vi "Generic Request (File).vi"(5 "method":string, 6 "timeout":i32=10000, 7 "output file":path, 8 "error in":errorcluster, 9 "file":path, 10 "url":string, 11 "Session In":refnum<class "Session.lvclass">) -> (0 "error out":errorcluster, 1 "body":string, 2 "headers":string, 3 "Session Out":refnum<class "Session.lvclass">, 4 "status code":u32)   [LabVIEW 2020, in "Library Commun.lvlib" / "Library Http.lvlib" / "Session.lvclass"]
uses:
  Session.lvclass
  Session.lvclass/Session.ctl
  lvwebclient_32.dll
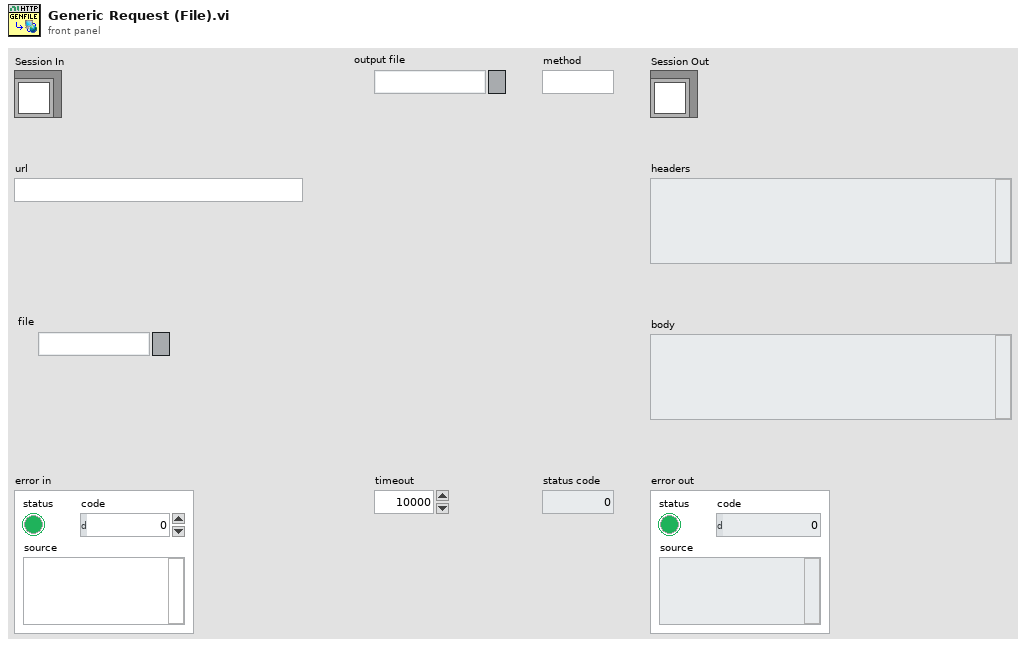
[diagram p1: front panel]
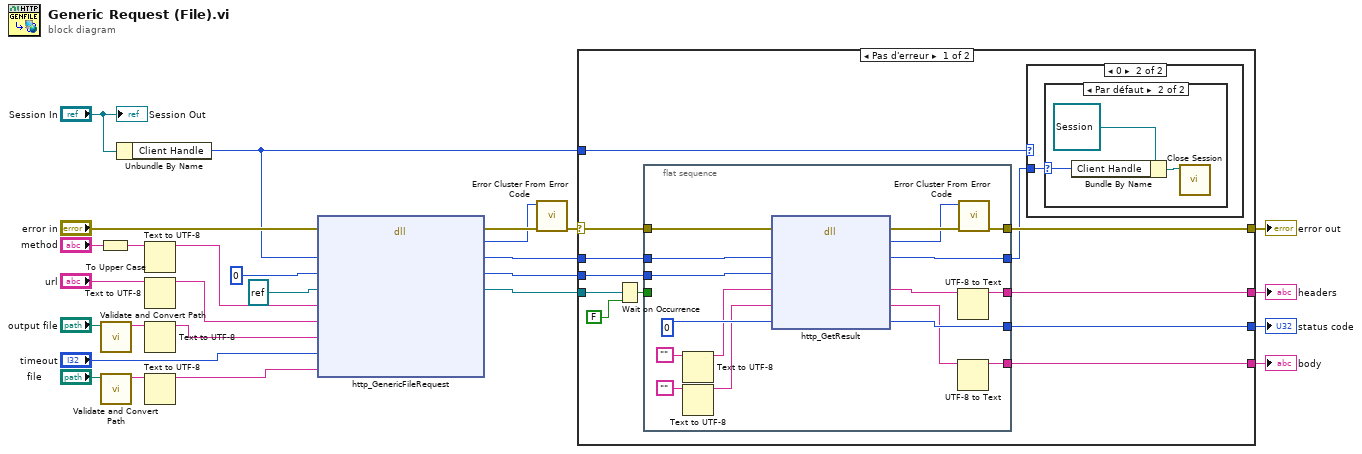
[diagram p0: block diagram]
diagram:
  n1 = To Upper Case(1:"method") -> (0:w16:string)
  n2 = call "Validate and Convert Path.vi"("path"="output file") -> ("validated path as string"=w19:string)  [unwired: 10 in]
  n3 = call "Validate and Convert Path.vi"("path"="file") -> ("validated path as string"=w2:string)  [unwired: 10 in]
  n4 = Unbundle By Name("Session In") -> ("Client Handle"=w9:u32)
  n5 = Text to UTF-8(11:w16) -> (3:w6:string)  [unwired: 2 in, 1 out]
  n6 = Text to UTF-8(11:"url") -> (3:w5:string)  [unwired: 2 in, 1 out]
  n7 = Text to UTF-8(11:w19) -> (3:w4:string)  [unwired: 2 in, 1 out]
  n8 = Text to UTF-8(11:w2) -> (3:w1:string)  [unwired: 2 in, 1 out]
  n9 = dll-call lib="C:/Users/ngarcin/OneDrive - Altyor/Standard TB/Class/Http Altyor/lvwebclient_*.*" fn="http_GenericFileRequest"(error in="error in", "handle"=w9, "request"=u32 0, "completeOccurrence"=refnum<k4> refnum ("occurrence"), "method"=w6, "url"=w5, "outPath"=w4, "timeoutInMs"="timeout", "requestBodyFile"=w1) -> (error out=w14:errorcluster, "return"=w13:i32, "handle"=w12:u32, "request"=w11:u32, "completeOccurrence"=w7:refnum<k4>)  [unwired: 7 in, 1 out]
  n10 = call <vilib>:"Error Cluster From Error Code.vi"("error in (no error)"=w14, "error code (0)"=w13) -> ("error out"=w27:errorcluster)  [unwired: 7 in]
  n11 = case shown="Pas d'erreur" w27 {
    selector: w27 -> [w37 w61]
    tunnel: w7 -> [w39 _]
    tunnel: w12 -> [w36 _]
    tunnel: w11 -> [w35 _]
    tunnel: [w34 _] -> w24
    tunnel: [w33 _] -> w23
    tunnel: [w32 _] -> w22
    tunnel: [w31 w61] -> w21
    tunnel: w9 -> [w30 _]
    frame No Error {
      n12 = Wait on Occurrence(1:FALSE, 2:w39) -> (0:w38:bool)  [unwired: 1 in]
      n13 = flat-sequence {
        tunnel: w38 -> [_]
        tunnel: w37 -> [w60]
        tunnel: w36 -> [w59]
        tunnel: w35 -> [w58]
        tunnel: [w56] -> w34
        tunnel: [w51] -> w33
        tunnel: [w50] -> w32
        tunnel: [w49] -> w31
        tunnel: [w48] -> w29
        frame #0 {
          n14 = Text to UTF-8(11:"") -> (3:w45:string)  [unwired: 2 in, 1 out]
          n15 = Text to UTF-8(11:"") -> (3:w44:string)  [unwired: 2 in, 1 out]
          n16 = dll-call lib="C:/Users/ngarcin/OneDrive - Altyor/Standard TB/Class/Http Altyor/lvwebclient_*.*" fn="http_GetResult"(error in=w60, "handle"=w59, "request"=w58, "returnHeader"=w45, "returnBody"=w44, "httpStatus"=u32 0) -> (error out=w55:errorcluster, "return"=w54:i32, "handle"=w48:u32, "returnHeader"=w53:string, "returnBody"=w52:string, "httpStatus"=w56:u32)  [unwired: 3 in, 1 out]
          n17 = UTF-8 to Text(11:w53) -> (3:w51:string)  [unwired: 2 in, 1 out]
          n18 = UTF-8 to Text(11:w52) -> (3:w50:string)  [unwired: 2 in, 1 out]
          n19 = call <vilib>:"Error Cluster From Error Code.vi"("error in (no error)"=w55, "error code (0)"=w54) -> ("error out"=w49:errorcluster)  [unwired: 7 in]
        }
      }
      n20 = case shown="0" w30 {
        tunnel: w29 -> [_ w40]
        frame Default {
        }
        frame 0 {
          n21 = case shown="Par défaut" w40 {
            selector: w40 -> [_ w43]
            frame 0 {
            }
            frame Default {
              n22 = Bundle By Name(cluster=refnum<class "Session.lvclass"> refnum ("NI_Advanced HTTP Client.lvlib:Session.lvclass"), "Client Handle"=w43) -> (w42:refnum<class "Session.lvclass">)
              n23 = call "Close Session.vi"("Session In"=w42) -> ()  [unwired: 10 in, 1 out]
            }
          }
        }
      }
    }
    frame Error {
    }
  }
  "error out" <- w21
  "headers" <- w23
  "body" <- w22
  "status code" <- w24
  "Session Out" <- "Session In"
